vi "QCP_Test.vi"() -> ()   [LabVIEW 2016]
uses:
  <userlib>/836-libraries/System/QCP_V2/QCPSupportCode/QCPData.ctl
  <userlib>/836-libraries/System/QCP_V2/QCPSupportCode/QCP_GetDblArr.vi
  <userlib>/836-libraries/System/QCP_V2/QCPSupportCode/QCP_GetDbl.vi
  <userlib>/836-libraries/System/QCP_V2/QCPSupportCode/QCP_SetDbl.vi
  <userlib>/836-libraries/System/QCP_V2/QCPSupportCode/QCP_SetDblArr.vi
panel:
  in  "Test To Run":enum32{"Basic Test", "Tuning Mode Test"}(tab)
  out "Value":dbl
  out "Value 2":dbl
  out "Values":dbl[](array[numeric])
  out "Values 2":dbl[](array[numeric])
  out "error out":errorcluster
  out "error out 2":errorcluster
  out "data value":T1
  in  "stop test":bool
  out "valOnePreTune":dbl
  out "valThreePreTune":dbl[](array[numeric])
  out "valSixPreTune":dbl[](array[numeric])
  out "valSixPostTune":dbl[](array[numeric])
  out "valThreePostTune":dbl[](array[numeric])
  out "valOnePostTune":dbl
  out "valOneDuringTune":dbl
  out "valThreeDuringTune":dbl[](array[numeric])
  out "valSixDuringTune":dbl[](array[numeric])
  in  "vaOneTune":dbl
  in  "valThreeTune":dbl[](array[numeric])
  in  "valSixTune":dbl[](array[numeric])
  out "error out 3":errorcluster
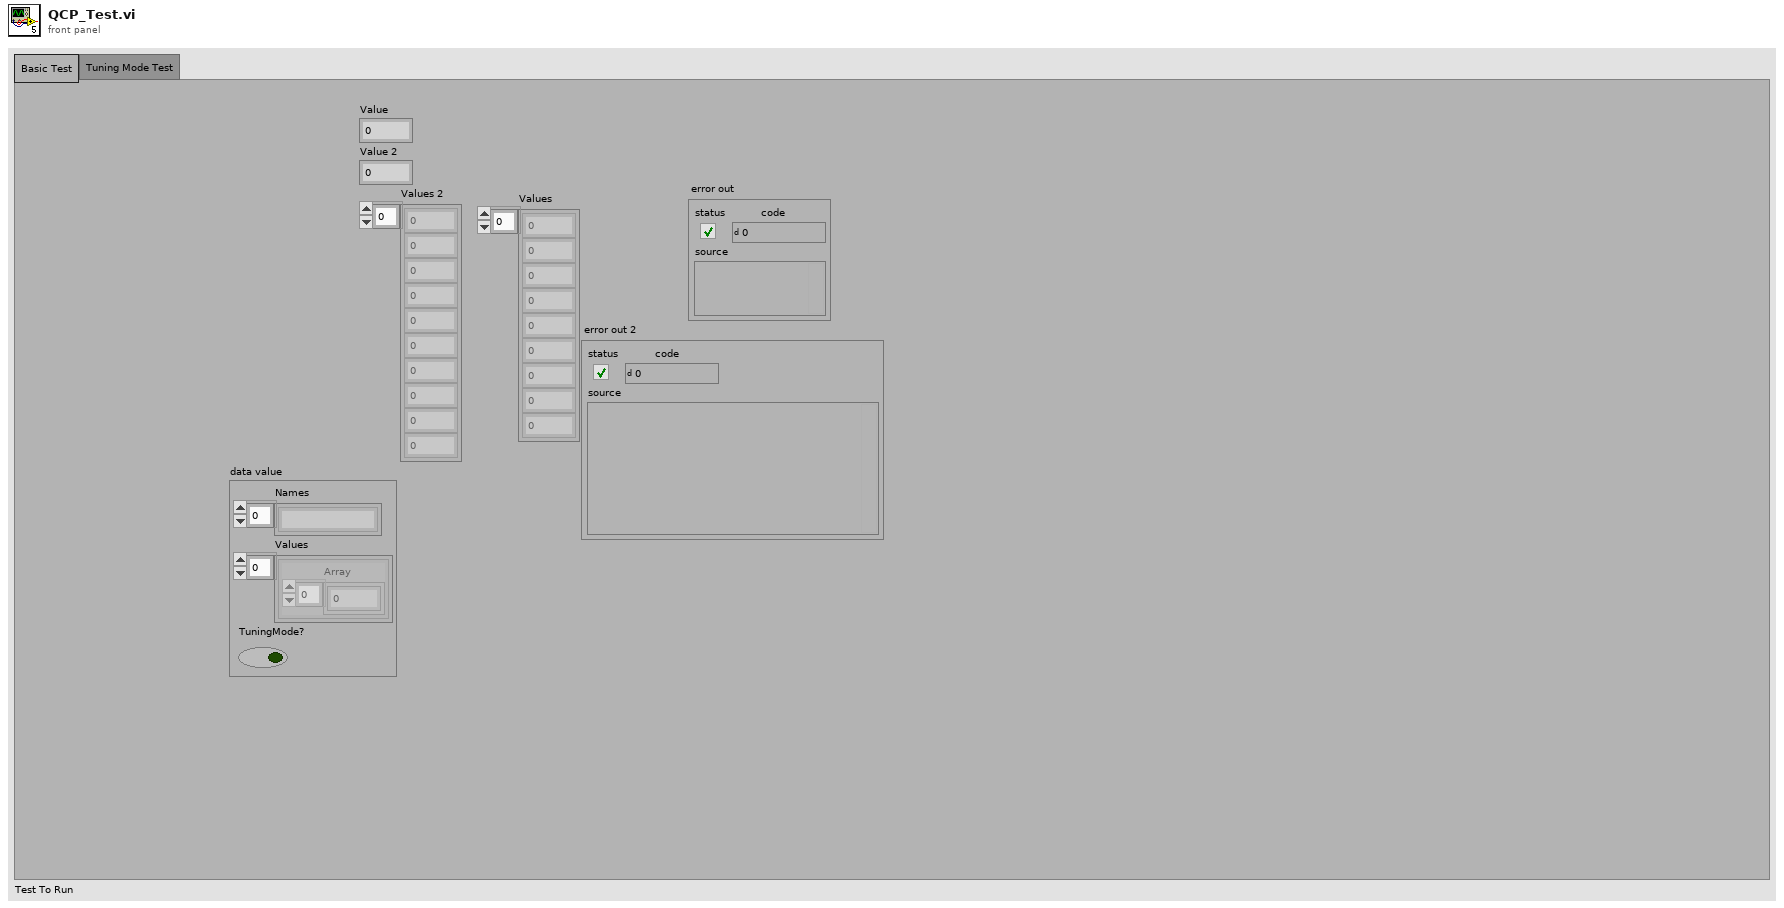
[diagram p1: front panel]
types:
  T1 = typedef "QCPData.ctl" = cluster{"Names":string[], "Values":cluster{"Array":dbl[]}[], "TuningMode?":bool}
  T2 = typedef "QCP_RefNum.ctl" = cluster{"Data Value Refnum":refnum<data-value>, "semaphore":T3}
  T3 = typedef "Semaphore RefNum" = refnum<k1>
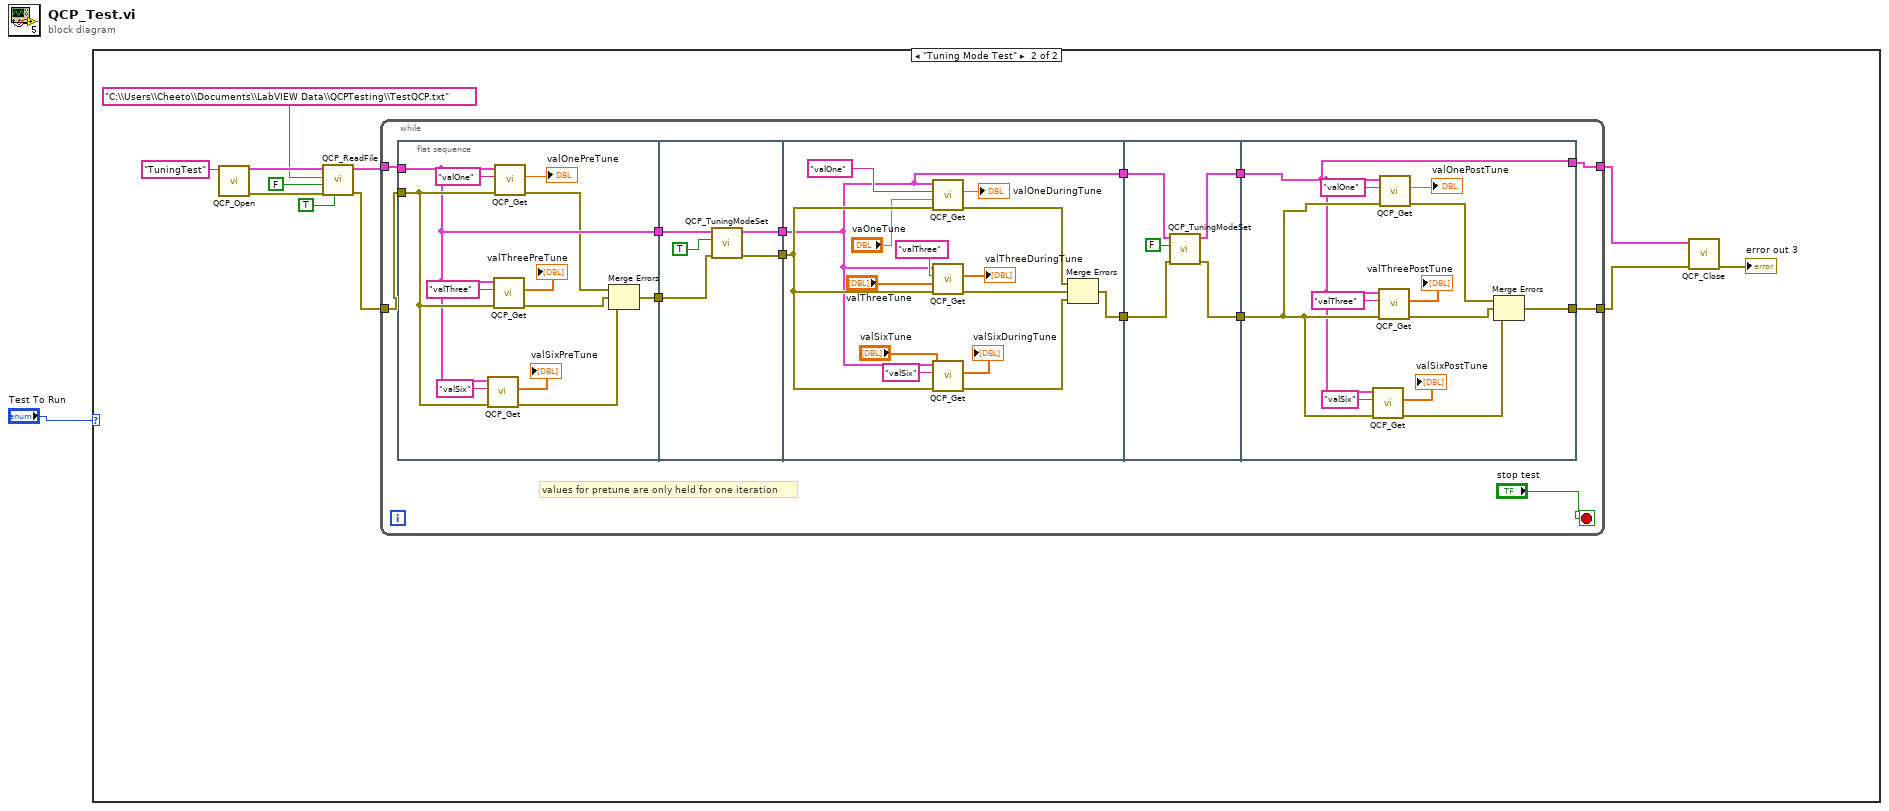
[diagram p0: block diagram]
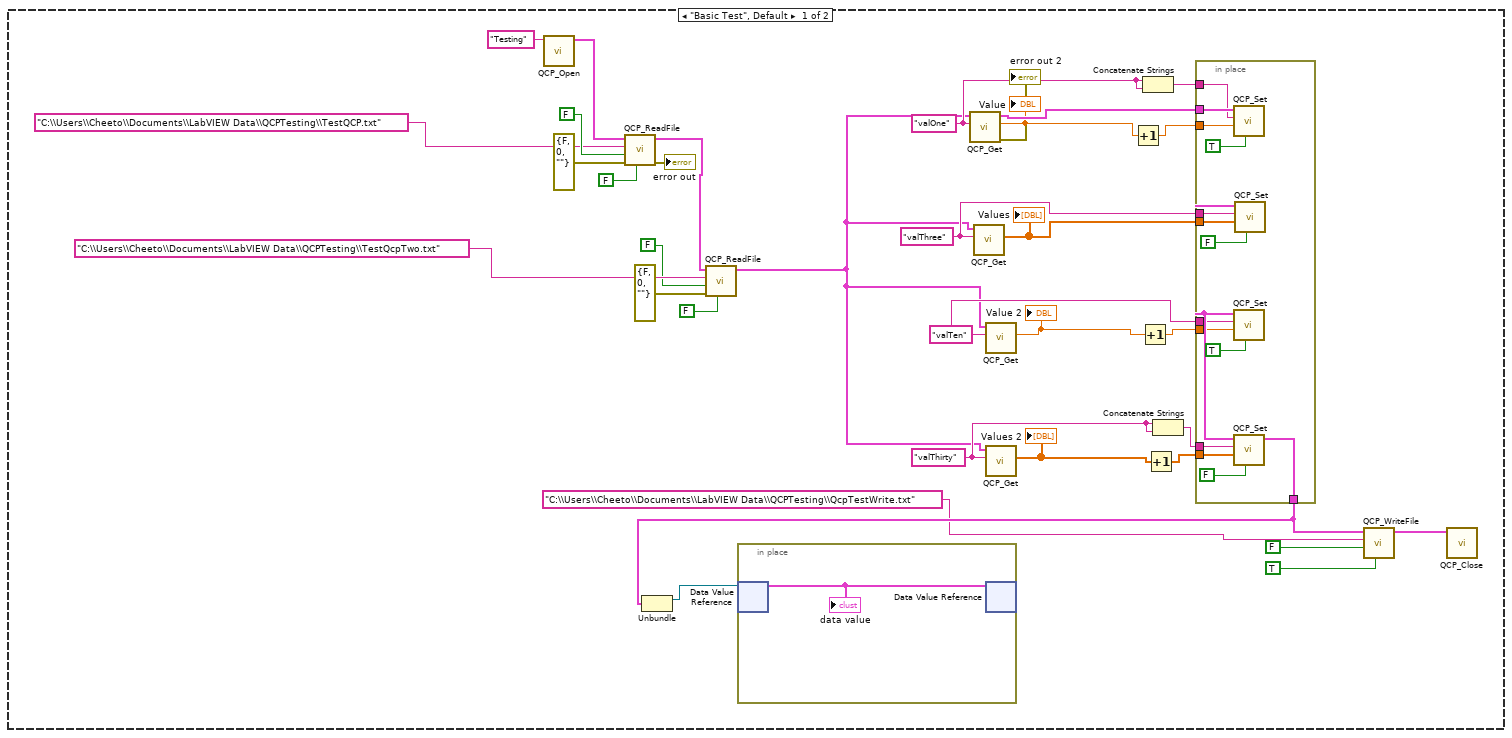
[diagram p2: hidden frame]
diagram:
  n1 = case shown="\"Tuning Mode Test\"" "Test To Run" {
    frame "Basic Test", Default {
      w17 = "valThree" ("Value Name")
      w11 = "valThirty" ("Value Name")
      w12 = "valTen" ("Value Name")
      w20 = "valOne" ("Value Name")
      n2 = call <userlib>:"QCP_Open.vi"("Name"="Testing") -> ("QCP_DevRef_Out"=w25:T2)  [unwired: 9 in, 1 out]
      n3 = call <userlib>:"QCP_ReadFile.vi"("Overrite Existing Data?"=FALSE, "error in"=errorcluster {"status"=FALSE, "code"=0, "source"=""}, "Path Relative?"=FALSE, "Path"="C:\\Users\\Cheeto\\Documents\\LabVIEW Data\\QCPTesting\\TestQCP.txt", "QCP_DevRef_In"=w25) -> ("error out"=→"error out":errorcluster, "QCP_DevRef_Out"=w24:T2)  [unwired: 5 in]
      n4 = call <userlib>:"QCP_ReadFile.vi"("Overrite Existing Data?"=FALSE, "error in"=errorcluster {"status"=FALSE, "code"=0, "source"=""}, "Path Relative?"=FALSE, "Path"="C:\\Users\\Cheeto\\Documents\\LabVIEW Data\\QCPTesting\\TestQcpTwo.txt", "QCP_DevRef_In"=w24) -> ("QCP_DevRef_Out"=w3:T2)  [unwired: 5 in, 1 out]
      n5 = call-poly <userlib>:"QCP_Get.vi"("Value Name"=w20, "QCP_DevRef_In"=w3) -> ("error out"=→"error out 2":errorcluster, "Value"=w22:dbl, "QCP_DevRef_Out"=w23:T2)  [unwired: 7 in]
      "Value" <- w22
      n6 = call-poly <userlib>:"QCP_Get.vi"("Value Name"=w17, "QCP_DevRef_In"=w3) -> ("Values"=w18:dbl[])  [unwired: 7 in, 2 out]
      "Values" <- w18
      n7 = call-poly <userlib>:"QCP_Get.vi"("Value Name"=w12, "QCP_DevRef_In"=w3) -> ("Value"=w16:dbl)  [unwired: 7 in, 2 out]
      "Value 2" <- w16
      n8 = call-poly <userlib>:"QCP_Get.vi"("Value Name"=w11, "QCP_DevRef_In"=w3) -> ("Values"=w14:dbl[])  [unwired: 7 in, 2 out]
      "Values 2" <- w14
      n9 = Increment(x=w22) -> (x+1=w21:dbl)
      n10 = Increment(x=w16) -> (x+1=w15:dbl)
      n11 = Concatenate Strings(w20, w20) -> (w19:string)
      n12 = Increment(x=w14) -> (x+1=w13:dbl[])
      n13 = Concatenate Strings(w11, w11) -> (w10:string)
      n14 = in-place {
        in-place-border: w23 -> [w49]
        in-place-border: w21 -> [w48]
        in-place-border: w19 -> [w47]
        in-place-border: w18 -> [w45]
        in-place-border: w17 -> [w43]
        in-place-border: w15 -> [w42]
        in-place-border: w13 -> [w41]
        in-place-border: w12 -> [w38]
        in-place-border: w10 -> [w37]
        in-place-border: [w36] -> w9
        n15 = call-poly <userlib>:"QCP_Set.vi"("Add if New?"=TRUE, "Value"=w48, "Name"=w47, "QCP_DevRef_In"=w49) -> ()  [unwired: 6 in, 2 out]
        n16 = call-poly <userlib>:"QCP_Set.vi"("Add if New?"=TRUE, "Value"=w42, "Name"=w38, "QCP_DevRef_In"=w49) -> ()  [unwired: 6 in, 2 out]
        n17 = call-poly <userlib>:"QCP_Set.vi"("Add if New?"=FALSE, "Values"=w41, "Name"=w37, "QCP_DevRef_In"=w49) -> ("QCP_DevRef_Out"=w36:T2)  [unwired: 6 in, 1 out]
        n18 = call-poly <userlib>:"QCP_Set.vi"("Add if New?"=FALSE, "Values"=w45, "Name"=w43, "QCP_DevRef_In"=w49) -> ()  [unwired: 6 in, 2 out]
      }
      n19 = Unbundle(w9) -> ("Data Value Refnum"=w27:refnum<data-value>)  [unwired: 1 out]
      n20 = in-place {
        n21 = in-place-dvr #1(w27) -> (w50:T1)  [unwired: 1 out]
        "data value" <- w50
        n22 = in-place-dvr #1(w50) -> ()  [unwired: 2 out]
      }
      n23 = call <userlib>:"QCP_WriteFile.vi"("Overrite?"=TRUE, "Path relative?"=FALSE, "Path"="C:\\Users\\Cheeto\\Documents\\LabVIEW Data\\QCPTesting\\QcpTestWrite.txt", "QCP_DevRef_In"=w9) -> ("QCP_DevRef_Out"=w5:T2)  [unwired: 6 in, 1 out]
      n24 = call <userlib>:"QCP_Close.vi"("QCP_DevRef_In"=w5) -> ()  [unwired: 10 in, 1 out]
    }
    frame "Tuning Mode Test" {
      n25 = call <userlib>:"QCP_Open.vi"("Name"="TuningTest") -> ("error out"=w59:errorcluster, "QCP_DevRef_Out"=w60:T2)  [unwired: 9 in]
      n26 = call <userlib>:"QCP_ReadFile.vi"("Overrite Existing Data?"=TRUE, "error in"=w59, "Path Relative?"=FALSE, "Path"="C:\\Users\\Cheeto\\Documents\\LabVIEW Data\\QCPTesting\\TestQCP.txt", "QCP_DevRef_In"=w60) -> ("error out"=w54:errorcluster, "QCP_DevRef_Out"=w55:T2)  [unwired: 5 in]
      n27 = while {
        tunnel: w54 -> [w65]
        tunnel: [w63] -> w52
        tunnel: w55 -> [w66]
        tunnel: [w64] -> w53
        stop <- "stop test" stop-if-true
        # "values for pretune are only held for one iteration"
        n28 = flat-sequence {
          tunnel: w66 -> [w79]
          tunnel: w65 -> [w83]
          tunnel: [w79] -> w74
          tunnel: [w75] -> w73
          tunnel: w74 -> [w91]
          tunnel: w73 -> [w89]
          tunnel: [w88] -> w72
          tunnel: [w87] -> w71
          tunnel: w72 -> [w106]
          tunnel: w71 -> [w96]
          tunnel: [w96] -> w70
          tunnel: [w92] -> w69
          tunnel: w70 -> [w109]
          tunnel: [w108] -> w68
          tunnel: w69 -> [w111]
          tunnel: [w110] -> w67
          tunnel: w68 -> [w112]
          tunnel: w67 -> [w114]
          tunnel: [w113] -> w63
          tunnel: [w112] -> w64
          frame #0 {
            n29 = call-poly <userlib>:"QCP_Get.vi"("error in (no error)"=w83, "Value Name"="valSix", "QCP_DevRef_In"=w79) -> ("error out"=w76:errorcluster, "Values"=→"valSixPreTune":dbl[])  [unwired: 6 in, 1 out]
            n30 = call-poly <userlib>:"QCP_Get.vi"("error in (no error)"=w83, "Value Name"="valThree", "QCP_DevRef_In"=w79) -> ("error out"=w77:errorcluster, "Values"=→"valThreePreTune":dbl[])  [unwired: 6 in, 1 out]
            n31 = call-poly <userlib>:"QCP_Get.vi"("error in (no error)"=w83, "Value Name"="valOne", "QCP_DevRef_In"=w79) -> ("error out"=w78:errorcluster, "Value"=→"valOnePreTune":dbl)  [unwired: 6 in, 1 out]
            n32 = Merge Errors(w78, w77, w76) -> (w75:errorcluster)
          }
          frame #1 {
            n33 = call <userlib>:"QCP_TuningModeSet.vi"("error in (no error)"=w89, "On?"=TRUE, "QCP_DevRef_In"=w91) -> ("error out"=w88:errorcluster, "QCP_DevRef_Out"=w87:T2)  [unwired: 7 in]
          }
          frame #2 {
            n34 = call-poly <userlib>:"QCP_Get.vi"("error in (no error)"=w106, "Tuning Value"="vaOneTune", "Value Name"="valOne", "QCP_DevRef_In"=w96) -> ("error out"=w95:errorcluster, "Value"=→"valOneDuringTune":dbl)  [unwired: 5 in, 1 out]
            n35 = call-poly <userlib>:"QCP_Get.vi"("error in (no error)"=w106, "Tuning Value"="valThreeTune", "Value Name"="valThree", "QCP_DevRef_In"=w96) -> ("error out"=w94:errorcluster, "Values"=→"valThreeDuringTune":dbl[])  [unwired: 5 in, 1 out]
            n36 = call-poly <userlib>:"QCP_Get.vi"("error in (no error)"=w106, "Tuning Value"="valSixTune", "Value Name"="valSix", "QCP_DevRef_In"=w96) -> ("error out"=w93:errorcluster, "Values"=→"valSixDuringTune":dbl[])  [unwired: 5 in, 1 out]
            n37 = Merge Errors(w95, w94, w93) -> (w92:errorcluster)
          }
          frame #3 {
            n38 = call <userlib>:"QCP_TuningModeSet.vi"("error in (no error)"=w111, "On?"=FALSE, "QCP_DevRef_In"=w109) -> ("error out"=w110:errorcluster, "QCP_DevRef_Out"=w108:T2)  [unwired: 7 in]
          }
          frame #4 {
            n39 = call-poly <userlib>:"QCP_Get.vi"("error in (no error)"=w114, "Value Name"="valSix", "QCP_DevRef_In"=w112) -> ("error out"=w115:errorcluster, "Values"=→"valSixPostTune":dbl[])  [unwired: 6 in, 1 out]
            n40 = call-poly <userlib>:"QCP_Get.vi"("error in (no error)"=w114, "Value Name"="valThree", "QCP_DevRef_In"=w112) -> ("error out"=w116:errorcluster, "Values"=→"valThreePostTune":dbl[])  [unwired: 6 in, 1 out]
            n41 = call-poly <userlib>:"QCP_Get.vi"("error in (no error)"=w114, "Value Name"="valOne", "QCP_DevRef_In"=w112) -> ("error out"=w117:errorcluster, "Value"=→"valOnePostTune":dbl)  [unwired: 6 in, 1 out]
            n42 = Merge Errors(w117, w116, w115) -> (w113:errorcluster)
          }
        }
      }
      n43 = call <userlib>:"QCP_Close.vi"("error in (no error)"=w52, "QCP_DevRef_In"=w53) -> ("error out"=→"error out 3":errorcluster)  [unwired: 9 in]
    }
  }
